vi "Set String.vi"(5 "use temporary file? (F)":bool, 8 "error in":errorcluster, 9 "value":string, 10 "variable name":string, 11 "GOLPI ref. in":T1={"pipe handle"={"lv_proc.dll file path"=path "", "process instance handle"=[], "debug mode"=FALSE, "debug data"=[]}, "fast read timeout [ms]"=500, "fast read settle time [ms]"=10, "fast read to multiple [ms]"=1, "max elements per input line"=100, "slow read timeout [ms]"=5000, "stdin double format specifier"="%_16e", "max elements per stdout output column"=100}) -> (0 "error out":errorcluster, 3 "GOLPI ref. out":T1={"pipe handle"={"lv_proc.dll file path"=path "", "process instance handle"=[], "debug mode"=FALSE, "debug data"=[]}, "fast read timeout [ms]"=500, "fast read settle time [ms]"=10, "fast read to multiple [ms]"=1, "max elements per input line"=100, "slow read timeout [ms]"=5000, "stdin double format specifier"="%_16e", "max elements per stdout output column"=100})   [LabVIEW 2013, in "GOLPI library.lvlib"]
doc: "Part of polymorph Set Variable.vi"
uses:
  GOLPI library.lvlib
  Type Definitions/GOLPI reference Type Def.ctl
  LV Process source distribution/Pipe Handle.ctl
  LV Process source distribution/LV Process library.lvlib
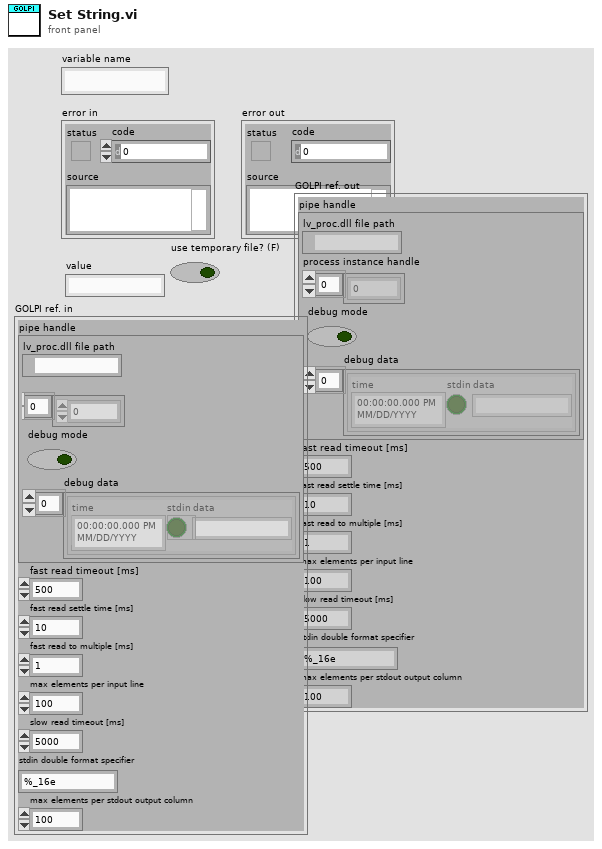
[diagram p1: front panel]
types:
  T1 = typedef "GOLPI library.lvlib/GOLPI reference Type Def.ctl" = cluster{"pipe handle":T2, "fast read timeout [ms]":u32, "fast read settle time [ms]":u32, "fast read to multiple [ms]":u32, "max elements per input line":u32, "slow read timeout [ms]":u32, "stdin double format specifier":string, "max elements per stdout output column":u32}
  T2 = typedef "LV Process library.lvlib/Pipe Handle.ctl" = cluster{"lv_proc.dll file path":path, "process instance handle":u32[], "debug mode":bool, "debug data":cluster{"time":timestamp, "stdin":bool, "data":string}[]}
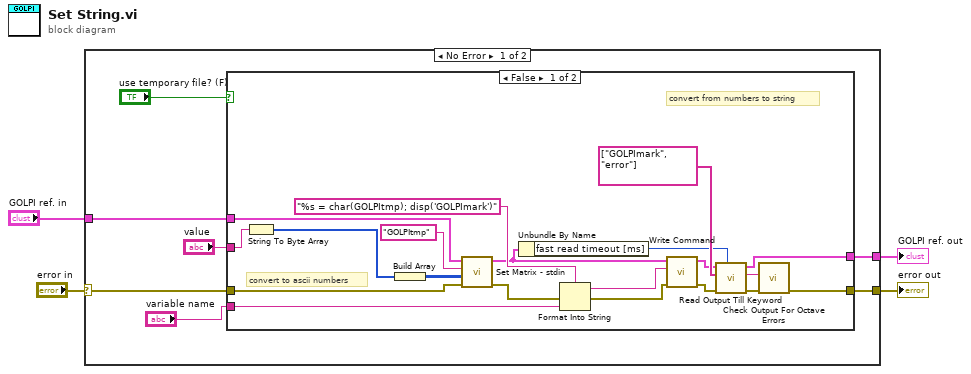
[diagram p0: block diagram]
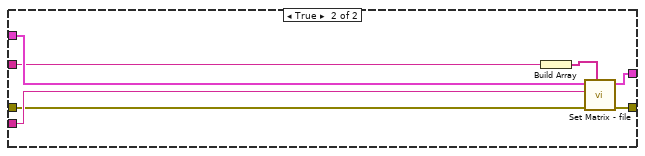
[diagram p2: hidden frame]
diagram:
  n1 = case shown="No Error" "error in" {
    selector: "error in" -> [w7 w40]
    tunnel: [w11 w40] -> w4
    tunnel: "GOLPI ref. in" -> [w6 w39]
    tunnel: [w10 w39] -> w1
    frame No Error {
      n2 = case shown="False" "use temporary file? (F)" {
        tunnel: [w31 w35] -> w11
        tunnel: [w30 w34] -> w10
        tunnel: "variable name" -> [w28 w38]
        tunnel: "value" -> [w18 w33]
        tunnel: w7 -> [w15 w36]
        tunnel: w6 -> [w14 w37]
        frame False {
          # "convert from numbers to string"
          # "convert to ascii numbers"
          n3 = String To Byte Array(string=w18) -> (unsigned byte array=w19:u8[])
          n4 = Build Array(w19) -> (w17:u8[][])
          n5 = call "Set Matrix - stdin.vi"("error in"=w15, "value"=w17, "variable name"="GOLPItmp", "GOLPI ref. in"=w14) -> ("error out"=w13:errorcluster, "GOLPI ref. out"=w12:T1)  [unwired: 6 in]
          n6 = Unbundle By Name(w12) -> ("fast read timeout [ms]"=w20:u32)
          n7 = Format Into String(format string="%s = char(GOLPItmp); disp('GOLPImark')", error in=w13, w28) -> (resulting string=w26:string, error out=w27:errorcluster)  [unwired: 1 in]
          n8 = call "Write Command.vi"("error in"=w27, "command"=w26, "GOLPI ref. in"=w12) -> ("error out"=w25:errorcluster, "GOLPI ref. out"=w22:T1)  [unwired: 7 in]
          n9 = call "Read Output Till Keyword.vi"("timeout [ms]"=w20, "error in"=w25, "keywords"=string[] ["GOLPImark", "error"], "GOLPI ref. in"=w22) -> ("error out"=w24:errorcluster, "read buffer"=w21:string, "GOLPI ref. out"=w30:T1)  [unwired: 4 in, 1 out]
          n10 = call "Check Output For Octave Errors.vi"("error in"=w24, "read buffer"=w21) -> ("error out"=w31:errorcluster)  [unwired: 9 in]
        }
        frame True {
          n11 = Build Array(w33) -> (w32:string[])
          n12 = call "Set Matrix - file.vi"("string array"=w32, "error in (no error)"=w36, "variable name"=w38, "GOLPI ref. in"=w37) -> ("error out"=w35:errorcluster, "GOLPI ref. out"=w34:T1)  [unwired: 6 in]
        }
      }
    }
    frame Error {
    }
  }
  "error out" <- w4
  "GOLPI ref. out" <- w1
